vi "2569 Switch Selection Dialog.vi"(8 "error in (no error)":errorcluster, 10 "NodeBroswerWF in":refnum<k24>(container), 11 "NIVS.System Definition Root":refnum<k24>) -> (0 "error out":errorcluster, 3 "NodeBrowserWF out":refnum<k24>)   [LabVIEW 2013]
doc: "Use this template to create a dialog box with event handling."
uses:
  NationalInstruments.VeriStand.SystemStorageUI
  NationalInstruments.VeriStand.SystemStorage
  NationalInstruments.VeriStand
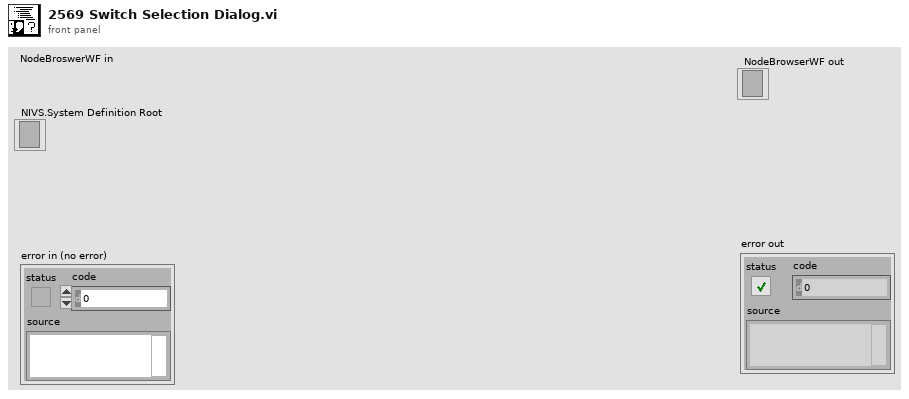
[diagram p1: front panel]
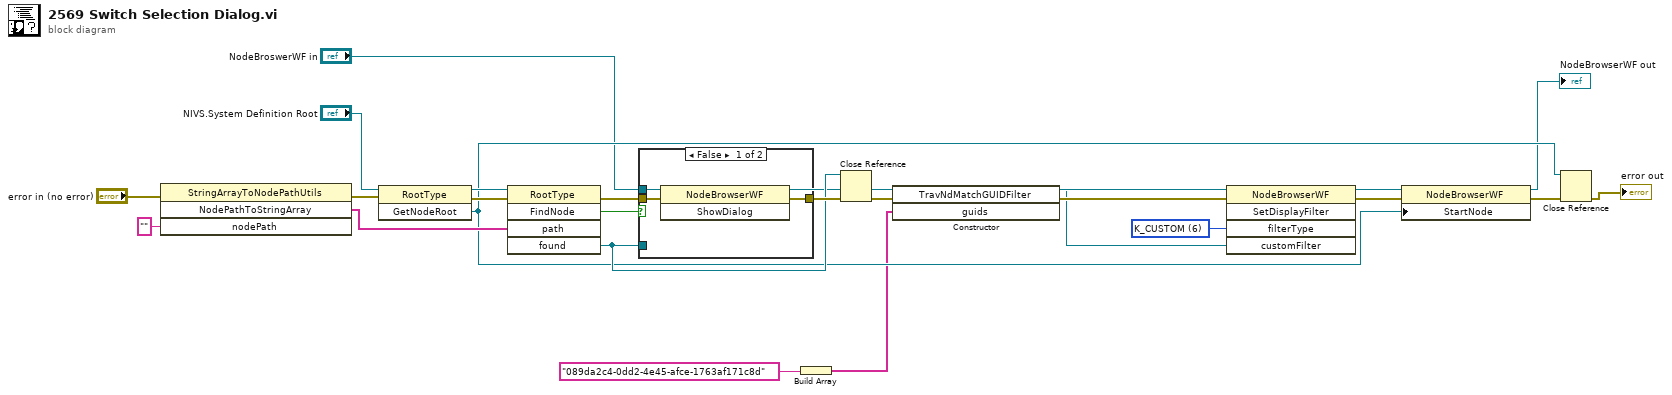
[diagram p0: block diagram]
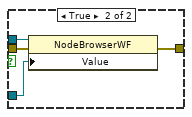
[diagram p2: hidden frame]
diagram:
  w8 = u8 6 items=["K_CHAN_R", "K_CHAN_W", "K_CHAN_RW", "K_CHAN_VOLT", "K_CHAN_FAULT", "K_ALL", "K_CUSTOM", "K_CHAN_R_VIS", "K_CHAN_W_VIS", "K_CHAN_RW_VIS", "K_CHAN_VOLT_VIS", "K_CHAN_FAULT_VIS", "K_WAVE", "K_WAVE_VIS", "K_WAVE_DBL", "K_WAVE_CDB", "K_WAVE_DBL_VIS", "K_WAVE_CDB_VIS"] ("filterType")
  n1 = invoke class="StringArrayToNodePathUtils" method="NodePathToStringArray"(error in="error in (no error)", "nodePath"="") -> (error out=w16:errorcluster, "NodePathToStringArray"=w15:string[])  [unwired: 2 in, 2 out]
  n2 = invoke class="RootType" method="GetNodeRoot"(reference="NIVS.System Definition Root", error in=w16) -> (reference out=w23:refnum<k24>, error out=w24:errorcluster, "GetNodeRoot"=w13:refnum<k24>)  [unwired: 1 in]
  n3 = invoke class="RootType" method="FindNode"(reference=w23, error in=w24, "path"=w15) -> (error out=w21:errorcluster, "FindNode"=w20:bool, "found"=w14:refnum<k24>)  [unwired: 2 in, 2 out]
  n4 = case shown="False" w20 {
    tunnel: w14 -> [_ w29]
    tunnel: w21 -> [w27 w30]
    tunnel: [w25 w28] -> w19
    tunnel: "NodeBroswerWF in" -> [w26 w31]
    frame False {
      n5 = invoke class="NodeBrowserWF" method="ShowDialog"(reference=w26, error in=w27) -> (error out=w25:errorcluster)  [unwired: 1 in, 2 out]
    }
    frame True {
      n6 = property class="NodeBrowserWF"(reference=w31, error in=w30, "Value"=w29) -> (error out=w28:errorcluster)  [unwired: 1 out]
    }
  }
  n7 = Build Array("089da2c4-0dd2-4e45-afce-1763af171c8d") -> (w9:string[])
  n8 = Close Reference(reference=w14, error in (no error)=w19) -> (error out=w7:errorcluster)
  n9 = constructor class="TravNdMatchGUIDFilter"(error in=w7, "guids"=w9) -> (reference out=w5:refnum<k24>, error out=w6:errorcluster)  [unwired: 2 in, 2 out]
  n10 = invoke class="NodeBrowserWF" method="SetDisplayFilter"(reference="NodeBroswerWF in", error in=w6, "filterType"=w8, "customFilter"=w5) -> (reference out=w11:refnum<k24>, error out=w4:errorcluster)  [unwired: 1 in, 3 out]
  n11 = property class="NodeBrowserWF"(reference=w11, error in=w4, "StartNode"=w13) -> (reference out=→"NodeBrowserWF out":refnum<k24>, error out=w22:errorcluster)
  n12 = Close Reference(reference=w13, error in (no error)=w22) -> (error out=→"error out":errorcluster)
